vi "Best y.vi"(7 "inimigos":bool, 8 "Ball false":dbl[](array[numeric]), 9 "Maior intervalo":bool, 10 "IA State":T2={"our_robots"=[], "enemy_robots"=[], "balls"=[], "geometry"={"line_width"=0, "field_length"=0, "field_width"=0, "boundary_width"=0, "referee_width"=0, "goal_width"=0, "goal_depth"=0, "goal_wall_width"=0, "center_circle_radius"=0, "defense_radius"=0, "defense_stretch"=0, "free_kick_from_defense_dist"=0, "penalty_spot_from_field_line_dist"=0, "penalty_line_from_spot_dist"=0}, "IA Judge"={"stage"="", "command"="", "our_goalie_id"=0.0, "enemy_goalie_id"=0.0, "command enum"=enum."Halt", "Time"=enum."Azul"}, "Received Timestamp"=timestamp(0 s since 1904-01-01), "Events"={"Touch"=FALSE, "Ball out"=FALSE, "id touch"=0.0, "Ball out of \nVision"=FALSE, "Ball inside \nGoalie area"=FALSE, "Robot not responding"=FALSE, "Robots responding status"=[1.0, 1.0, 1.0, 1.0, 1.0, 1.0], "Enemy Ball \nPossession"=FALSE, "Pass State"=FALSE, "id end of pass"=0.0, "Kick"=FALSE, "Id ini Possession"=0.0, "Ball Possesion"=FALSE, "Id Possesion"=0.0}}, 11 "Best y para varredura?":bool) -> (2 "Best y":dbl, 3 "Gap kick":dbl, 4 "Eclipse":bool, 5 "Gap Coord":dbl[](array[numeric]))   [LabVIEW 2017]
uses:
  Core/AI Input.ctl
  Core/AI Robot.ctl
  Intel/Functions Enum.ctl
  Intel/AttackerStates.ctl
  Core/AI Ball.ctl
  Core/Field Size.ctl
  Core/AI Judge.ctl
  Intel/Command Enum.ctl
  Events/Events.ctl
  segment.ctl
  <vilib>/Analysis/baseanly.llb/Real Dot Product.vi
  <vilib>/Analysis/NI_AALBase.lvlib
panel:
  out "Vetor de gaps \ncorreto":T1[](array[typedef])
  out "Vetor de gaps":T1[](array[typedef])
  in  "eclipse angle eps":dbl=0.035 format="%#_13g"
  out "pilha output (merged)":T1[](array[typedef])
  out "Vetor de segmentos ordenado":T1[](array[typedef])
  out "Vetor de segmentos (sombras)":T1[](array[typedef])
  # "Maior ângulo"
  # "amigos"
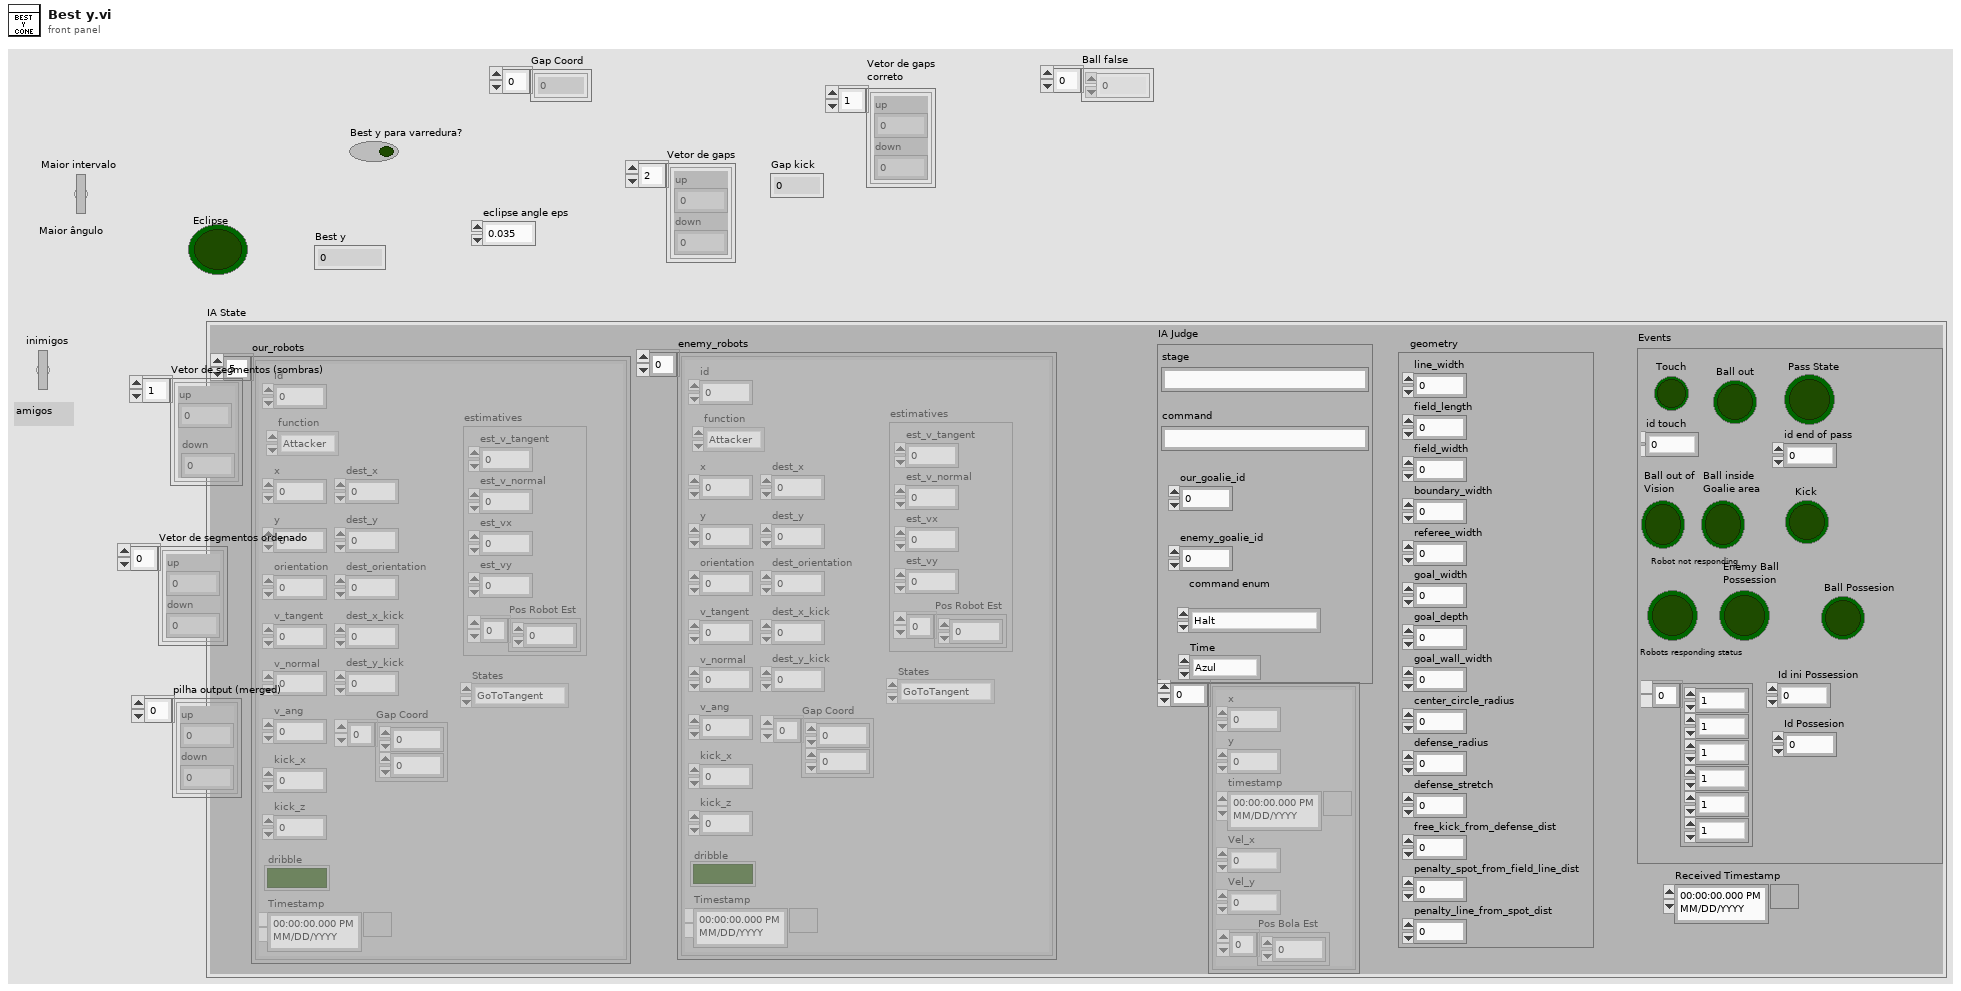
[diagram p1: front panel]
types:
  T1 = typedef "segment.ctl" = cluster{"up":dbl, "down":dbl}
  T2 = typedef "AI Input.ctl" = cluster{"our_robots":T3[], "enemy_robots":T3[], "balls":T6[], "geometry":T7, "IA Judge":T8, "Received Timestamp":timestamp, "Events":T10}
  T3 = typedef "AI Robot.ctl" = cluster{"id":u32, "function":T4, "x":dbl, "y":dbl, "orientation":dbl, "v_tangent":dbl, "v_normal":dbl, "v_ang":dbl, "kick_x":dbl, "kick_z":dbl, "dribble":bool, "Timestamp":timestamp, "dest_x":dbl, "dest_y":dbl, "dest_orientation":dbl, "estimatives":cluster{"est_v_tangent":dbl, "est_v_normal":dbl, "est_vx":dbl, "est_vy":dbl, "Pos Robot Est":dbl[]}, "dest_x_kick":dbl, "dest_y_kick":dbl, "Gap Coord":dbl[], "States":T5}
  T4 = typedef "Functions Enum.ctl" = enum16{"Attacker", "Goalie", "Defender", "Striker", "Goto 0", "Dummy", "Kicker", "ZigZag"}
  T5 = typedef "AttackerStates.ctl" = enum16{"Pass", "GoToTangent", "BallGetting", "GoToKick", ""}
  T6 = typedef "AI Ball.ctl" = cluster{"x":dbl, "y":dbl, "timestamp":timestamp, "Vel_x":dbl, "Vel_y":dbl, "Pos Bola Est":dbl[]}
  T7 = typedef "Field Size.ctl" = cluster{"line_width":u32, "field_length":u32, "field_width":u32, "boundary_width":u32, "referee_width":u32, "goal_width":u32, "goal_depth":u32, "goal_wall_width":u32, "center_circle_radius":u32, "defense_radius":u32, "defense_stretch":u32, "free_kick_from_defense_dist":u32, "penalty_spot_from_field_line_dist":u32, "penalty_line_from_spot_dist":u32}
  T8 = typedef "AI Judge.ctl" = cluster{"stage":string, "command":string, "our_goalie_id":dbl, "enemy_goalie_id":dbl, "command enum":T9, "Time":enum16{"Azul", "Amarelo"}}
  T9 = typedef "Command Enum.ctl" = enum16{"Halt", "Stop", "Force Start", "PKA Normal Start", "Prepare Kickoff Ally", "PKE Normal Start", "Prepare Kickoff Enemy", "Prepare Penalty Ally", "PPA Normal Start", "Prepare Penalty Enemy", "PPE Normal Start", "Direct Free Enemy", "Direct Free Ally", "Indirect Free Enemy", "Indirect Free Ally", "Timeout Enemy", "Timeout Ally", "Goal Enemy", "Goal Ally", "Ball Placement Enemy", "Ball Placement Ally", "Normal Half Time", "Extra Time Break", "Extra Half Time", "None", "Post Game"}
  T10 = typedef "Events.ctl" = cluster{"Touch":bool, "Ball out":bool, "id touch":dbl, "Ball out of \nVision":bool, "Ball inside \nGoalie area":bool, "Robot not responding":bool, "Robots responding status":dbl[], "Enemy Ball \nPossession":bool, "Pass State":bool, "id end of pass":dbl, "Kick":bool, "Id ini Possession":dbl, "Ball Possesion":bool, "Id Possesion":dbl}
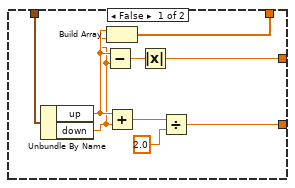
[diagram p4: hidden frame]
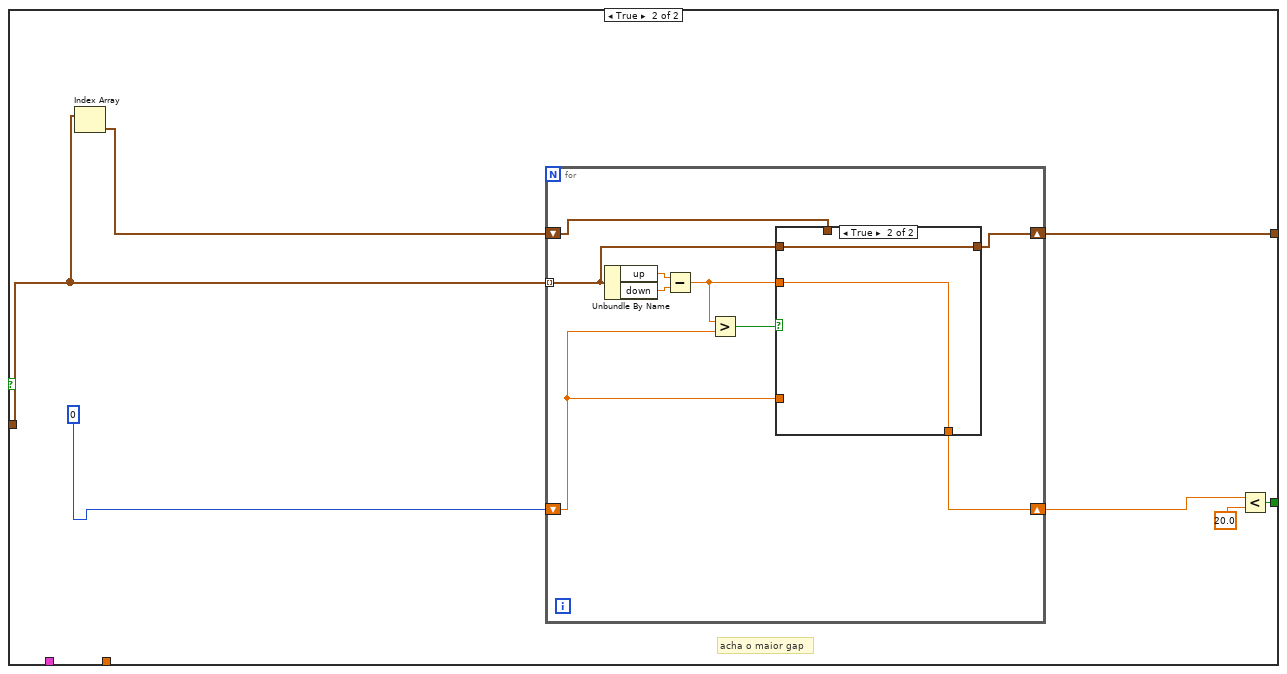
[diagram p7: hidden frame]
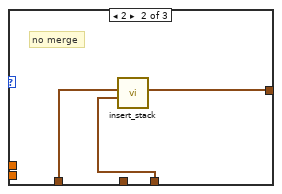
[diagram p9: hidden frame]
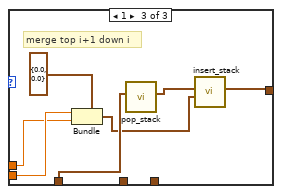
[diagram p10: hidden frame]
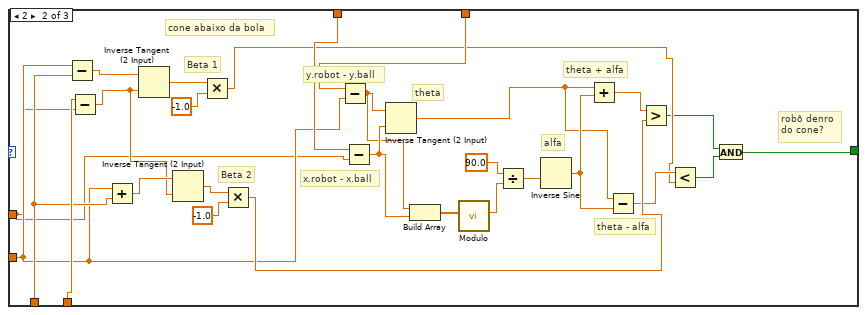
[diagram p12: hidden frame]
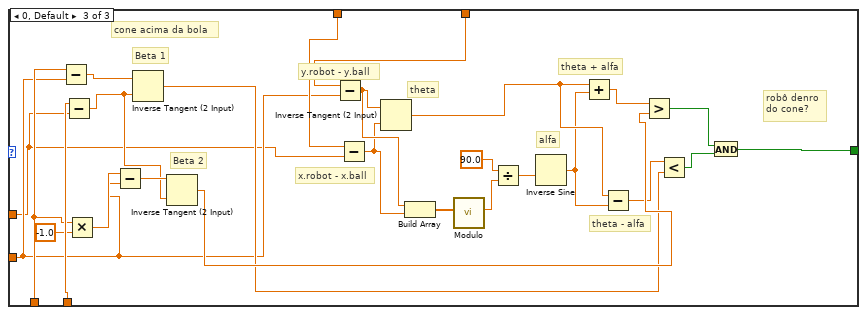
[diagram p13: hidden frame]
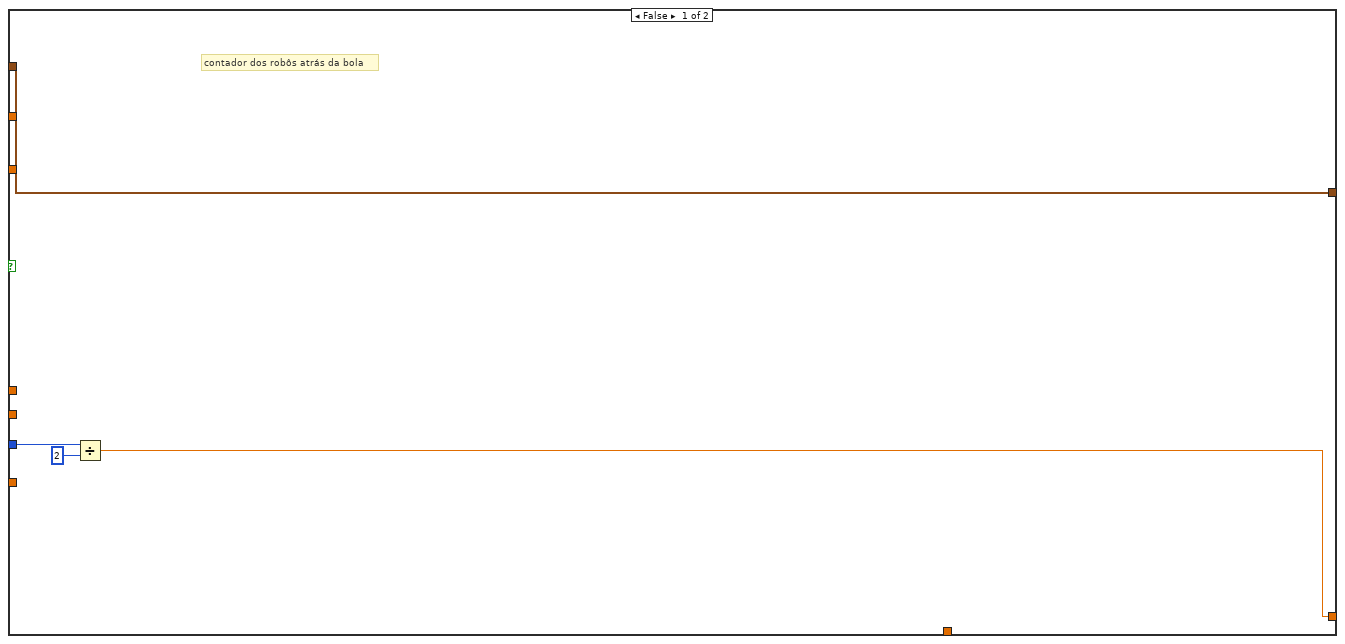
[diagram p14: hidden frame]
diagram:
  w16 = T6 {"x"=0.0, "y"=0.0, "timestamp"=timestamp(0 s since 1904-01-01), "Vel_x"=0.0, "Vel_y"=0.0, "Pos Bola Est"=[]} ("element")
  # "goal_width/2"
  # "field_length/2"
  # "balls"
  # "vetor de gaps"
  # "upper"
  n1 = Unbundle By Name("IA State") -> ("enemy_robots"=w25:T3[], "our_robots"=w24:T3[])
  n2 = Unbundle By Name("IA State") -> ("balls"=w18:T6[], "geometry.field_length"=w44:u32, "geometry.goal_width"=w41:u32)
  n3 = Select(t=w25, s="inimigos", f=w24) -> (s? t:f=w23:T3[])
  n4 = Divide(x=w41, y=u32 2 ("x")) -> (x/y=w5:dbl)
  n5 = Index Array(array=w18) -> (element=w17:T6)  [unwired: 1 in]
  n6 = Index Array(array="Ball false") -> (element #1=w21:dbl, element #2=w20:dbl)  [unwired: 2 in]
  n7 = Bundle By Name(cluster=w16, "x"=w21, "y"=w20) -> ()  [unwired: 1 out]
  n8 = case shown="False" "Best y para varredura?" {
    tunnel: [w46 w47] -> w15
    tunnel: w17 -> [w46 _]
    tunnel: w16 -> [_ w47]
    frame False {
    }
    frame True {
    }
  }
  n9 = for {
    shift-right: [w81] -> w28
    shift-left: T1[] [] -> [w80]
    tunnel: w44 -> [w57]
    tunnel: w5 -> [w59]
    tunnel: w5 -> [w78]
    shift-right: [w77] -> w26
    shift-left: _ -> [_]
    tunnel: w23 -> [w76] mode=indexing
    tunnel: "inimigos" -> [w74]
    tunnel: w15 -> [w51]
    # "y ball"
    # "x ball"
    # "y.robot"
    # "x.robot"
    # "field_length/2"
    # "goal_width/2"
    # "y ball"
    # "x ball"
    n10 = Unbundle By Name(w76) -> ("x"=w55:dbl, "y"=w54:dbl)
    n11 = Multiply(x=w55, y=-1.0) -> (x*y=w73:dbl)
    n12 = Unbundle By Name(w51) -> ("x"=w50:dbl, "y"=w48:dbl)
    n13 = Absolute Value(x=w50) -> (abs(x)=w72:dbl)
    n14 = Absolute Value(x=w55) -> (abs(x)=w79:dbl)
    n15 = Select(t=w55, s=w74, f=w73) -> (s? t:f=w52:dbl)
    n16 = Greater?(x=w79, y=w72) -> (0:w71:bool)
    n17 = Multiply(x=w59, y=-1.0) -> (x*y=w63:dbl)
    n18 = Greater?(x=w48, y=w59) -> (0:w62:bool)
    n19 = Less?(x=w48, y=w63) -> (x < y?=w61:bool)
    n20 = Select(t=1, s=w62, f=0) -> (s? t:f=w69:i32)
    n21 = Select(t=0, s=w61, f=1) -> (s? t:f=w70:i32)
    n22 = Add(x=w69, y=w70) -> (x+y=w60:i32)
    n23 = Divide(x=w57, y=2.0) -> (x/y=w56:dbl)
    n24 = case shown="1" w60 {
      tunnel: w59 -> [w84 w110 w158]
      tunnel: w56 -> [w105 w130 w160]
      tunnel: w52 -> [w92 w117 w153]
      tunnel: w54 -> [w91 w118 w154]
      tunnel: [w93 w119 w144] -> w49
      tunnel: w50 -> [w82 w108 w136]
      tunnel: w48 -> [w83 w109 w137]
      frame 1 {
        # "robô denro\ndo cone?"
        # "cone centrado"
        # "theta - alfa"
        # "theta + alfa"
        # "theta"
        # "alfa"
        # "x.robot - x.ball"
        # "y.robot - y.ball"
        # "Beta 2"
        # "Beta 1"
        n25 = Subtract(x=w84, y=w83) -> (x-y=w106:dbl)
        n26 = Subtract(x=w105, y=w82) -> (x-y=w107:dbl)
        n27 = Add(x=w83, y=w84) -> (x+y=w104:dbl)
        n28 = Inverse Tangent (2 Input)(1:w107, 2:w106) -> (0:w87:dbl)
        n29 = Inverse Tangent (2 Input)(1:w107, 2:w104) -> (0:w103:dbl)
        n30 = Multiply(x=w103, y=-1.0) -> (x*y=w89:dbl)
        n31 = Subtract(x=w91, y=w83) -> (x-y=w94:dbl)
        n32 = Subtract(x=w92, y=w82) -> (x-y=w95:dbl)
        n33 = Inverse Tangent (2 Input)(1:w95, 2:w94) -> (0:w100:dbl)
        n34 = Build Array(w94, w95) -> (w96:dbl[])
        n35 = call "Modulo.vi"("2D vector"=w96) -> ("Modulo"=w97:dbl)  [unwired: 10 in]
        n36 = Divide(x=90.0, y=w97) -> (x/y=w98:dbl)
        n37 = Inverse Sine(1:w98) -> (0:w101:dbl)
        n38 = Add(x=w100, y=w101) -> (x+y=w90:dbl)
        n39 = Subtract(x=w100, y=w101) -> (x-y=w88:dbl)
        n40 = Greater?(x=w90, y=w89) -> (0:w85:bool)
        n41 = Less?(x=w88, y=w87) -> (x < y?=w86:bool)
        n42 = And(x=w85, y=w86) -> (x .and. y?=w93:bool)
      }
      frame 2 {
        # "robô denro\ndo cone?"
        # "cone abaixo da bola"
        # "theta - alfa"
        # "theta + alfa"
        # "theta"
        # "alfa"
        # "x.robot - x.ball"
        # "y.robot - y.ball"
        # "Beta 2"
        # "Beta 1"
        n43 = Subtract(x=w109, y=w110) -> (x-y=w132:dbl)
        n44 = Subtract(x=w130, y=w108) -> (x-y=w131:dbl)
        n45 = Add(x=w109, y=w110) -> (x+y=w133:dbl)
        n46 = Inverse Tangent (2 Input)(1:w131, 2:w132) -> (0:w128:dbl)
        n47 = Inverse Tangent (2 Input)(1:w131, 2:w133) -> (0:w134:dbl)
        n48 = Multiply(x=w128, y=-1.0) -> (x*y=w113:dbl)
        n49 = Multiply(x=w134, y=-1.0) -> (x*y=w115:dbl)
        n50 = Subtract(x=w118, y=w109) -> (x-y=w120:dbl)
        n51 = Subtract(x=w117, y=w108) -> (x-y=w121:dbl)
        n52 = Inverse Tangent (2 Input)(1:w121, 2:w120) -> (0:w126:dbl)
        n53 = Build Array(w120, w121) -> (w122:dbl[])
        n54 = call "Modulo.vi"("2D vector"=w122) -> ("Modulo"=w123:dbl)  [unwired: 10 in]
        n55 = Divide(x=90.0, y=w123) -> (x/y=w124:dbl)
        n56 = Inverse Sine(1:w124) -> (0:w127:dbl)
        n57 = Add(x=w126, y=w127) -> (x+y=w116:dbl)
        n58 = Subtract(x=w126, y=w127) -> (x-y=w114:dbl)
        n59 = Greater?(x=w116, y=w115) -> (0:w111:bool)
        n60 = Less?(x=w114, y=w113) -> (x < y?=w112:bool)
        n61 = And(x=w111, y=w112) -> (x .and. y?=w119:bool)
      }
      frame 0, Default {
        # "robô denro\ndo cone?"
        # "cone acima da bola"
        # "theta - alfa"
        # "theta + alfa"
        # "theta"
        # "alfa"
        # "x.robot - x.ball"
        # "y.robot - y.ball"
        # "Beta 2"
        # "Beta 1"
        n62 = Subtract(x=w158, y=w137) -> (x-y=w161:dbl)
        n63 = Subtract(x=w160, y=w136) -> (x-y=w155:dbl)
        n64 = Multiply(x=w158, y=-1.0) -> (x*y=w157:dbl)
        n65 = Subtract(x=w157, y=w137) -> (x-y=w156:dbl)
        n66 = Inverse Tangent (2 Input)(1:w155, 2:w161) -> (0:w139:dbl)
        n67 = Inverse Tangent (2 Input)(1:w155, 2:w156) -> (0:w142:dbl)
        n68 = Subtract(x=w154, y=w137) -> (x-y=w152:dbl)
        n69 = Subtract(x=w153, y=w136) -> (x-y=w151:dbl)
        n70 = Inverse Tangent (2 Input)(1:w151, 2:w152) -> (0:w146:dbl)
        n71 = Build Array(w152, w151) -> (w150:dbl[])
        n72 = call "Modulo.vi"("2D vector"=w150) -> ("Modulo"=w149:dbl)  [unwired: 10 in]
        n73 = Divide(x=90.0, y=w149) -> (x/y=w148:dbl)
        n74 = Inverse Sine(1:w148) -> (0:w145:dbl)
        n75 = Add(x=w146, y=w145) -> (x+y=w143:dbl)
        n76 = Subtract(x=w146, y=w145) -> (x-y=w140:dbl)
        n77 = Greater?(x=w143, y=w142) -> (0:w141:bool)
        n78 = Less?(x=w140, y=w139) -> (x < y?=w138:bool)
        n79 = And(x=w141, y=w138) -> (x .and. y?=w144:bool)
      }
    }
    n80 = And(x=w71, y=w49) -> (x .and. y?=w53:bool)
    n81 = case shown="True" w53 {
      tunnel: [w165 w172] -> w81
      tunnel: w80 -> [w165 w174]
      tunnel: w57 -> [w164 w179]
      tunnel: w59 -> [_ w178]
      tunnel: w78 -> [_ w171]
      tunnel: [w162 w170] -> w77
      tunnel: w54 -> [_ w169]
      tunnel: w52 -> [_ w168]
      tunnel: w50 -> [_ w166]
      tunnel: w48 -> [_ w167]
      frame False {
        # "contador dos robôs atrás da bola"
        n82 = Divide(x=w164, y=u32 2) -> (x/y=w162:dbl)
      }
      frame True {
        n83 = flat-sequence {
          tunnel: w169 -> [w214]
          tunnel: w179 -> [w210]
          tunnel: w178 -> [w195]
          tunnel: [w185] -> w177
          tunnel: [w184] -> w176
          tunnel: [w196] -> w175
          tunnel: w174 -> [w189]
          tunnel: [w189] -> w173
          tunnel: [w183] -> w170
          tunnel: w168 -> [w182]
          tunnel: w167 -> [w180]
          tunnel: w166 -> [w181]
          tunnel: w177 -> [w218]
          tunnel: w176 -> [w217]
          tunnel: w175 -> [w219]
          tunnel: w173 -> [w220]
          tunnel: [w216] -> w172
          tunnel: w171 -> [w215]
          frame #0 {
            # "theta - alfa"
            # "alfa + theta"
            # "theta"
            # "alfa"
            # "x.robot - x.ball"
            # "y.robot - y.ball"
            n84 = Divide(x=w210, y=u32 2 ("x")) -> (x/y=w183:dbl)
            n85 = Subtract(x=w182, y=w181) -> (x-y=w193:dbl)
            n86 = Subtract(x=w214, y=w180) -> (x-y=w194:dbl)
            n87 = Multiply(x=w195, y=-1.0) -> (x*y=w201:dbl)
            n88 = Subtract(x=w183, y=w181) -> (x-y=w186:dbl)
            n89 = Inverse Tangent (2 Input)(1:w193, 2:w194) -> (0:w192:dbl)
            n90 = Build Array(w194, w193) -> (w213:dbl[])
            n91 = call "Modulo.vi"("2D vector"=w213) -> ("Modulo"=w211:dbl)  [unwired: 10 in]
            n92 = Divide(x=90.0, y=w211) -> (x/y=w191:dbl)
            n93 = Inverse Sine(1:w191) -> (0:w190:dbl)
            n94 = Subtract(x=w192, y=w190) -> (x-y=w206:dbl)
            n95 = Tangent(1:w206) -> (0:w205:dbl)
            n96 = Add(x=w192, y=w190) -> (x+y=w208:dbl)
            n97 = Tangent(1:w208) -> (0:w207:dbl)
            n98 = Multiply(x=w205, y=w186) -> (x*y=w187:dbl)
            n99 = Multiply(x=w207, y=w186) -> (x*y=w188:dbl)
            n100 = Add(x=w187, y=w180) -> (x+y=w184:dbl)
            n101 = Add(x=w188, y=w180) -> (x+y=w185:dbl)
            n102 = Less?(x=w185, y=w201) -> (x < y?=w200:bool)
            n103 = Less?(x=w184, y=w201) -> (x < y?=w199:bool)
            n104 = Greater?(x=w184, y=w195) -> (0:w203:bool)
            n105 = Greater?(x=w185, y=w195) -> (0:w204:bool)
            n106 = And(x=w204, y=w203) -> (x .and. y?=w198:bool)
            n107 = And(x=w200, y=w199) -> (x .and. y?=w197:bool)
            n108 = Or(x=w198, y=w197) -> (x .or. y?=w196:bool)
          }
          frame #1 {
            # "goal_width/2"
            n109 = case shown="False" w219 {
              tunnel: [w229 w232] -> w216
              tunnel: w220 -> [w228 w232]
              tunnel: w218 -> [w227 _]
              tunnel: w217 -> [w225 _]
              tunnel: w215 -> [w224 _]
              frame False {
                n110 = Max & Min(x=w227, y=w224) -> (min(x,y)=w226:dbl)  [unwired: 1 out]
                n111 = Multiply(x=w224, y=-1.0) -> (x*y=w222:dbl)
                n112 = Max & Min(x=w225, y=w222) -> (max(x,y)=w221:dbl)  [unwired: 1 out]
                n113 = Bundle(cluster=T1 {"up"=0.0, "down"=0.0} ("segment 2"), "up"=w226, "down"=w221) -> (w230:T1)
                n114 = Insert Into Array(array=w228, new element=w230) -> (w229:T1[])  [unwired: 1 in]
              }
              frame True {
              }
            }
          }
        }
      }
    }
  }
  "Vetor de segmentos (sombras)" <- w28
  n115 = Sort 1D Array(array=w28) -> (sorted array=w40:T1[])
  "Vetor de segmentos ordenado" <- w40
  n116 = Index Array(array=w40) -> (element=w39:T1)  [unwired: 1 in]
  n117 = call "insert_stack.vi"("novo elemento"=w39, "pilha input"=T1[] []) -> ("pilha output"=w37:T1[])  [unwired: 9 in]
  n118 = for {
    shift-right: [w233] -> w36
    shift-left: w37 -> [w235]
    tunnel: w40 -> [w234] mode=indexing
    i -> [w236]
    n119 = case shown="Default" w236 {
      tunnel: w235 -> [w240 w268]
      tunnel: w234 -> [w243 _]
      tunnel: [w241 w268] -> w233
      frame Default {
        # "pilha"
        # "i+1"
        # "i"
        # "i+1"
        # "i"
        n120 = call "top_stack.vi"("pilha input"=w240) -> ("top"=w242:T1)  [unwired: 10 in]
        n121 = Unbundle By Name(w242) -> ("up"=w239:dbl, "down"=w244:dbl)
        n122 = Unbundle By Name(w243) -> ("down"=w238:dbl, "up"=w245:dbl)
        n123 = Greater Or Equal?(x=w238, y=w239) -> (x >= y?=w237:bool)
        n124 = Less?(x=w238, y=w244) -> (x < y?=w247:bool)
        n125 = Select(t=1, s=w237, f=0) -> (s? t:f=w249:i32)
        n126 = Select(t=0, s=w247, f=1) -> (s? t:f=w248:i32)
        n127 = Add(x=w249, y=w248) -> (x+y=w246:i32)
        n128 = case shown="0, Default" w246 {
          tunnel: w245 -> [_ _ w266]
          tunnel: w244 -> [_ _ w265]
          tunnel: w242 -> [_ _ _]
          tunnel: w243 -> [w254 w259 _]
          tunnel: [w257 w258 w261] -> w241
          tunnel: w240 -> [w256 w260 w264]
          frame 0, Default {
            # "merge:  i+1"
            n129 = call "pop_stack.vi"("pilha input"=w256) -> ("pilha output"=w255:T1[])  [unwired: 9 in]
            n130 = call "insert_stack.vi"("novo elemento"=w254, "pilha input"=w255) -> ("pilha output"=w257:T1[])  [unwired: 9 in]
          }
          frame 2 {
            # "no merge"
            n131 = call "insert_stack.vi"("novo elemento"=w259, "pilha input"=w260) -> ("pilha output"=w258:T1[])  [unwired: 9 in]
          }
          frame 1 {
            # "merge top i+1 down i"
            n132 = Bundle(cluster=T1 {"up"=0.0, "down"=0.0} ("segment 2"), "up"=w266, "down"=w265) -> (w262:T1)
            n133 = call "pop_stack.vi"("pilha input"=w264) -> ("pilha output"=w263:T1[])  [unwired: 9 in]
            n134 = call "insert_stack.vi"("novo elemento"=w262, "pilha input"=w263) -> ("pilha output"=w261:T1[])  [unwired: 9 in]
          }
        }
      }
      frame 0 {
      }
    }
  }
  "pilha output (merged)" <- w36
  n135 = Reverse 1D Array(array=w36) -> (reversed array=w35:T1[])
  n136 = for {
    tunnel: w35 -> [w276] mode=indexing
    shift-right: [w270] -> w32
    shift-left: T1[] [] -> [w272]
    shift-right: [w271] -> w31
    shift-left: w5 -> [w273]
    n137 = Unbundle By Name(w276) -> ("up"=w269:dbl, "down"=w271:dbl)
    n138 = Bundle(cluster=T1 {"up"=0.0, "down"=0.0} ("segment 2"), "up"=w273, "down"=w269) -> (w275:T1)
    n139 = Insert Into Array(array=w272, new element=w275) -> (w270:T1[])  [unwired: 1 in]
  }
  n140 = Multiply(x=w5, y=-1.0) -> (x*y=w29:dbl)
  n141 = Bundle(cluster=T1 {"up"=0.0, "down"=0.0} ("segment 2"), "up"=w31, "down"=w29) -> (w34:T1)
  n142 = Insert Into Array(array=w32, new element=w34) -> (w6:T1[])  [unwired: 1 in]
  n143 = Array Size(array=w6) -> (size(s)=w8:i32)
  n144 = Decrement(x=w8) -> (x-1=w7:i32)
  n145 = for {
    N: w7 -> [_]
    shift-right: [w277] -> w4
    shift-left: w6 -> [w279]
    i -> [w278]
    n146 = Increment(x=w278) -> (x+1=w287:i32)
    n147 = Index Array(array=w279, index=w278) -> (element=w280:T1)
    n148 = Index Array(array=w279, index=w287) -> (element=w286:T1)
    n149 = Unbundle By Name(w286) -> ("up"=w284:dbl, "down"=w281:dbl)
    n150 = Unbundle By Name(w280) -> ("up"=w282:dbl, "down"=w285:dbl)
    n151 = Equal?(x=w285, y=w284) -> (x = y?=w283:bool)
    n152 = case shown="True" w283 {
      tunnel: w282 -> [_ w297]
      tunnel: w281 -> [_ w296]
      tunnel: w280 -> [_ w295]
      tunnel: w279 -> [w288 w293]
      tunnel: w278 -> [_ w290]
      tunnel: [w288 w289] -> w277
      frame False {
      }
      frame True {
        n153 = Bundle By Name(cluster=w295, "up"=w297, "down"=w296) -> (w291:T1)
        n154 = Delete From Array(array=w293, length=2, index=w290) -> (array with subset deleted=w292:T1[])  [unwired: 1 out]
        n155 = Insert Into Array(array=w292, index=w290, new element=w291) -> (w289:T1[])
      }
    }
  }
  "Vetor de gaps" <- w4
  n156 = for {
    tunnel: w5 -> [w307]
    tunnel: w4 -> [w300] mode=indexing
    shift-right: [w302] -> w1
    shift-left: T1[] [] -> [w301]
    n157 = Unbundle By Name(w300) -> ("up"=w299:dbl, "down"=w298:dbl)
    n158 = Multiply(x=w307, y=-1.0) -> (x*y=w306:dbl)
    n159 = Greater?(x=w299, y=w307) -> (0:w304:bool)
    n160 = Less?(x=w298, y=w306) -> (x < y?=w303:bool)
    n161 = Or(x=w304, y=w303) -> (x .or. y?=w305:bool)
    n162 = case shown="False" w305 {
      tunnel: [w309 w312] -> w302
      tunnel: w301 -> [w309 w313]
      tunnel: w299 -> [_ w310]
      tunnel: w298 -> [_ w311]
      frame True {
      }
      frame False {
        n163 = Bundle(cluster=T1 {"up"=0.0, "down"=0.0} ("segment 2"), "up"=w310, "down"=w311) -> (w314:T1)
        n164 = Insert Into Array(array=w313, new element=w314) -> (w312:T1[])  [unwired: 1 in]
      }
    }
  }
  "Vetor de gaps \ncorreto" <- w1
  n165 = case shown="False" "Maior intervalo" {
    tunnel: [w318 w356] -> w12
    tunnel: [w317 w354] -> w13
    tunnel: w1 -> [w324 w355]
    tunnel: w15 -> [w316 _]
    tunnel: w26 -> [w321 _]
    frame False {
      # "acha o maior ângulo"
      n166 = Unbundle By Name(w316) -> ("x"=w323:dbl, "y"=w322:dbl)
      n167 = Index Array(array=w324) -> (element=w325:T1)  [unwired: 1 in]
      n168 = for {
        tunnel: w324 -> [w346] mode=indexing
        shift-right: [w347] -> w320
        shift-left: 0 -> [w329]
        shift-right: [w345] -> w317
        shift-left: w325 -> [w344]
        tunnel: w323 -> [w328]
        tunnel: w322 -> [w327]
        tunnel: w321 -> [w343]
        # "theta"
        # "cos (theta)"
        # "vetor bola-down"
        # "vetor bola-up"
        n169 = Unbundle By Name(w346) -> ("up"=w342:dbl, "down"=w339:dbl)
        n170 = Subtract(x=w343, y=w328) -> (x-y=w340:dbl)
        n171 = Subtract(x=w339, y=w327) -> (x-y=w338:dbl)
        n172 = Subtract(x=w342, y=w327) -> (x-y=w341:dbl)
        n173 = Build Array(w340, w338) -> (w336:dbl[])
        n174 = Build Array(w340, w341) -> (w337:dbl[])
        n175 = call-poly <vilib>:"Dot Product.vi"("Y Vector"=w336, "X Vector"=w337) -> ("X * Y"=w333:dbl)  [unwired: 1 out]
        n176 = call "Modulo.vi"("2D vector"=w337) -> ("Modulo"=w335:dbl)  [unwired: 10 in]
        n177 = call "Modulo.vi"("2D vector"=w336) -> ("Modulo"=w334:dbl)  [unwired: 10 in]
        n178 = Multiply(x=w335, y=w334) -> (x*y=w332:dbl)
        n179 = Divide(x=w333, y=w332) -> (x/y=w331:dbl)
        n180 = Inverse Cosine(1:w331) -> (0:w330:dbl)
        n181 = Greater?(x=w330, y=w329) -> (0:w348:bool)
        n182 = case shown="True" w348 {
          tunnel: w330 -> [_ w352]
          tunnel: [w349 w352] -> w347
          tunnel: w346 -> [_ w351]
          tunnel: [w350 w351] -> w345
          tunnel: w344 -> [w350 _]
          tunnel: w329 -> [w349 _]
          frame False {
          }
          frame True {
          }
        }
      }
      n183 = Less?(x=w320, y="eclipse angle eps") -> (x < y?=w318:bool)
    }
    frame True {
      # "acha o maior gap"
      n184 = Index Array(array=w355) -> (element=w358:T1)  [unwired: 1 in]
      n185 = for {
        tunnel: w355 -> [w363] mode=indexing
        shift-right: [w364] -> w357
        shift-left: 0 -> [w361]
        shift-right: [w362] -> w354
        shift-left: w358 -> [w360]
        n186 = Unbundle By Name(w363) -> ("up"=w368:dbl, "down"=w367:dbl)
        n187 = Subtract(x=w368, y=w367) -> (x-y=w365:dbl)
        n188 = Greater?(x=w365, y=w361) -> (0:w366:bool)
        n189 = case shown="True" w366 {
          tunnel: w365 -> [_ w372]
          tunnel: [w370 w372] -> w364
          tunnel: w363 -> [_ w371]
          tunnel: [w369 w371] -> w362
          tunnel: w361 -> [w370 _]
          tunnel: w360 -> [w369 _]
          frame False {
          }
          frame True {
          }
        }
      }
      n190 = Less?(x=w357, y=20.0) -> (x < y?=w356:bool)
    }
  }
  n191 = case shown="True" w12 {
    selector: w12 -> [_ w387]
    tunnel: w13 -> [w379 _]
    tunnel: [w378 w384] -> w9
    tunnel: [w376 0.0] -> w10
    tunnel: [w373 dbl[] [0.0, 0.0] ("Gap Coord")] -> w11
    frame False {
      n192 = Unbundle By Name(w379) -> ("up"=w375:dbl, "down"=w374:dbl)
      n193 = Subtract(x=w375, y=w374) -> (x-y=w377:dbl)
      n194 = Build Array(w375, w374) -> (w373:dbl[])
      n195 = Add(x=w375, y=w374) -> (x+y=w380:dbl)
      n196 = Absolute Value(x=w377) -> (abs(x)=w376:dbl)
      n197 = Divide(x=w380, y=2.0) -> (x/y=w378:dbl)
    }
    frame True {
      n198 = Multiply(x=1.0, y=0.0) -> (x*y=w384:dbl)
      "Eclipse" <- w387
    }
  }
  "Best y" <- w9
  "Gap kick" <- w10
  "Gap Coord" <- w11
